vi "DropDown VI Wrapper Testing.vi"(7 "Software Config File Path":path) -> ()   [LabVIEW 2016]
uses:
  DropDown VI Wrapper Type Defs/Drop Down Bar.ctl
  <vilib>/Utility/miscctls.llb/LVPointTypeDef.ctl
  <vilib>/Utility/miscctls.llb/LVRectTypeDef.ctl
panel:
  in  "Visible Two":bool
  in  "Visible":bool
  in  "Screen and Exit Bar":T1
  in  "Drop Down Control 1":T2
  in  "Drop Down Control 2":T2
  in  "Drop Down Control 3":T2
  in  "Drop Down Control 4":T2
  in  "Drop Down Control 5":T2
  in  "Drop Down Control 6":T2
  in  "Drop Down Control 7":T2
  in  "Drop Down Control 8":T2
  in  "Drop Down Control 9":T2
  in  "Drop Down Control 10":T2
  # "Some Text"
  # "Some Text"
  # "Some Text"
  # "Some Text"
  # "Some Text"
  # "Some Text"
  # "Some Text"
  # "Some Text"
  # "Some Text"
  # "Some Text"
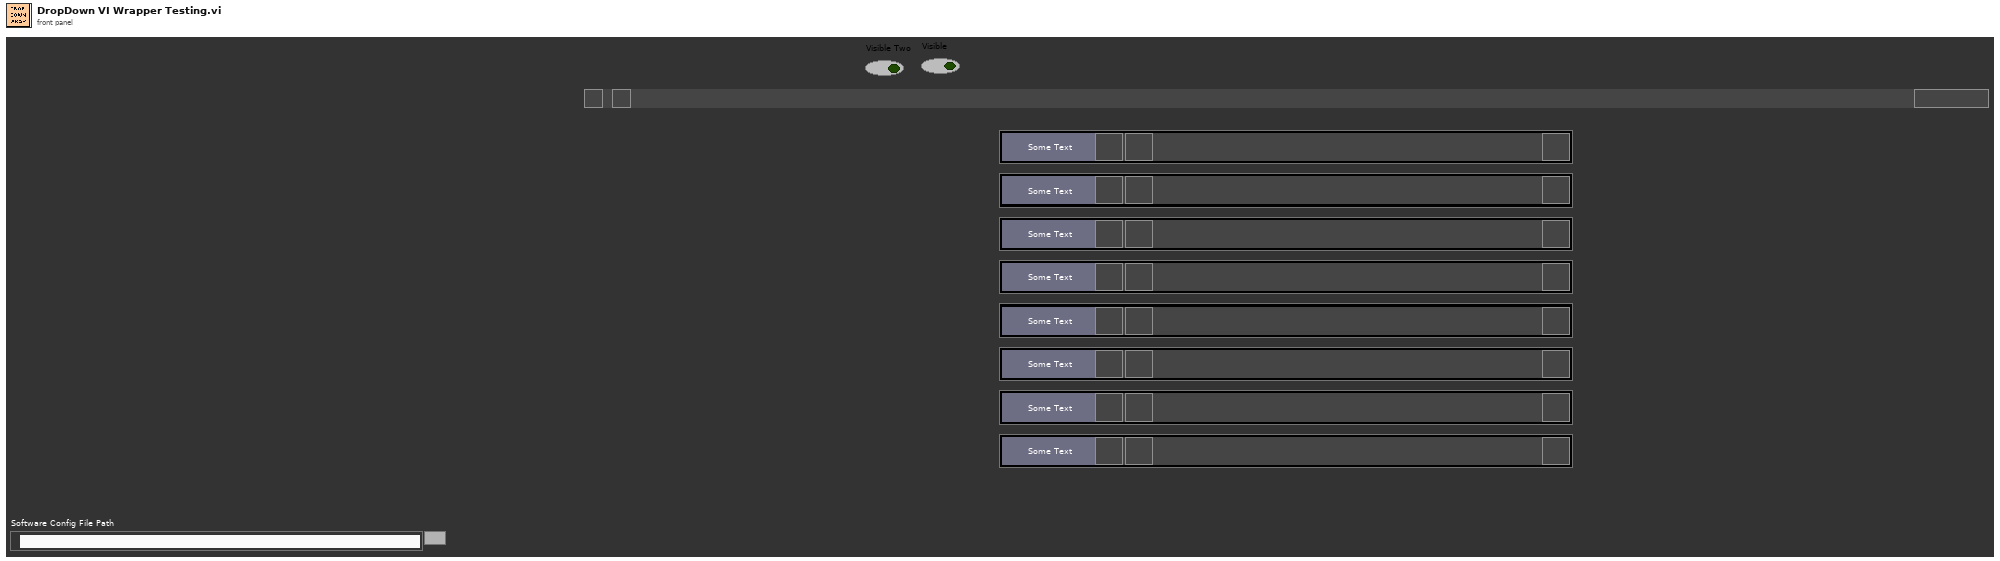
[diagram p1: front panel]
types:
  T1 = cluster{"Max Left":bool, "Max Right":bool, "Exit":bool, "Messages":string}
  T2 = typedef "Drop Down Bar.ctl" = cluster{"Right Width":bool, "Messages":string, "Abort VI":bool, "Close VI":bool}
  T3 = enum16{"Always On", "Always Off", "Off While Running"}
  T4 = typedef "LVPointTypeDef.ctl" = cluster{"Horizontal":i16, "Vertical":i16}
  T5 = enum32{"Invalid", "Standard", "Closed", "Hidden", "Minimized", "Maximized"}
  T6 = typedef "LVRectTypeDef.ctl" = cluster{"Left":i16, "Top":i16, "Right":i16, "Bottom":i16}
  T7 = enum8{"Enabled", "Disabled", "Disabled and Grayed Out"}
  T8 = cluster{"VI Path":path, "VI Refnum":refnum<vi>}[]
  T9 = typedef "lveventtype.ctl" = enum32{"Null", "Timeout", "Annotation Menu Selection", "Annotation Menu Selection?", "App Instance Close", "App Instance Close?", "Autoscale Range Change", "Bookmark Info Change", "Cell Edit", "Cell Edit?", "Cursor Grab", "Cursor Grab?", "Cursor Menu Selection", "Cursor Menu Selection?", "Cursor Move", "Cursor Release", "Data Change", "Direction Change", "Display State Change", "Drag Ended", "Drag Enter", "Drag Leave", "Drag Over", "Drag Source Update", "Drag Starting", "Drag Starting?", "Drop", "Exec State Change", "Key Down", "Key Down?", "Key Repeat", "Key Repeat?", "Key Up", "Listbox Double Click", "Menu Activation?", "Menu Selection (App)", "Menu Selection? (App)", "Menu Selection (User)", "Mouse Down", "Mouse Down?", "Mouse Enter", "Mouse Leave", "Mouse Move", "Mouse Up", "Mouse Wheel", "NI Security User Change (App)", "Pane Size", "Panel Close", "Panel Close?", "Panel Resize", "Plot Attribute Change", "Scale Range Change", "Shortcut Menu Activation?", "Shortcut Menu Selection (App)", "Shortcut Menu Selection? (App)", "Shortcut Menu Selection (User)", "Tree Double Click", "Tree Drag", "Tree Drag?", "Tree Drop", "Tree Drop?", "Tree Item Close", "Tree Item Close?", "Tree Item Open", "Tree Item Open?", "User Event", "Value Change"}
  T10 = typedef "LVAllMonitorsDisplayTypeDef.ctl" = cluster{"Bounds":cluster{"Left":i16, "Top":i16, "Right":i16, "Bottom":i16}, "Depth":i16}[]
  T11 = cluster{"Bounds":cluster{"Left":i16, "Top":i16, "Right":i16, "Bottom":i16}, "Depth":i16}
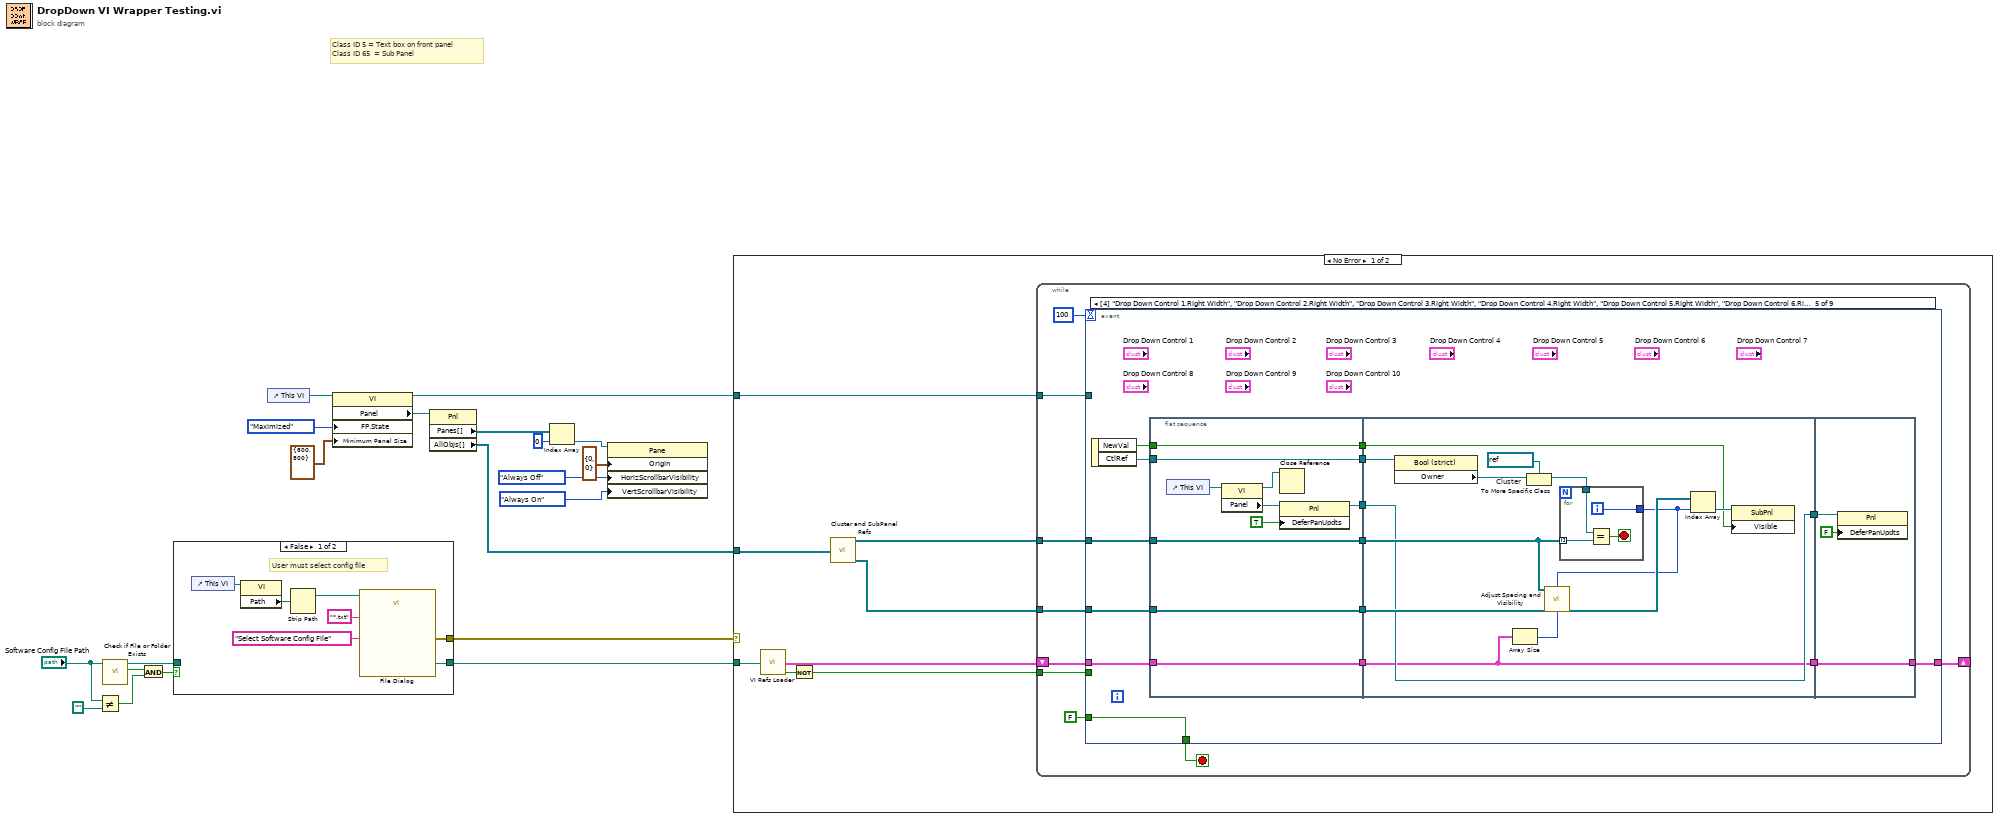
[diagram p0: block diagram]
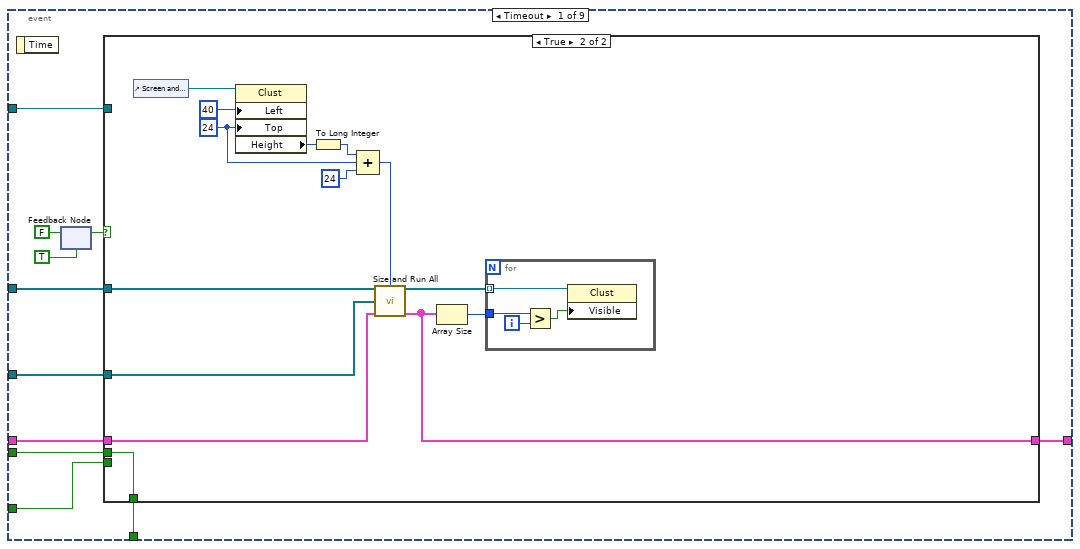
[diagram p2: hidden frame]
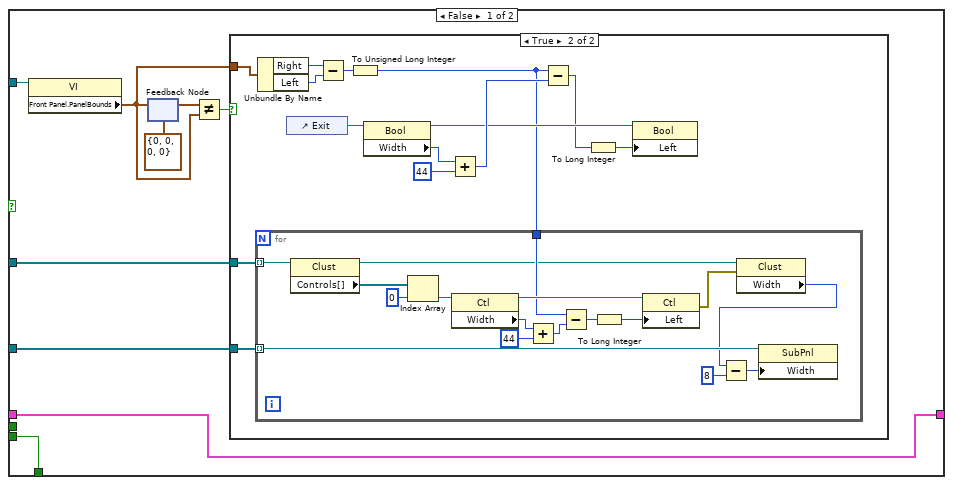
[diagram p3: hidden frame]
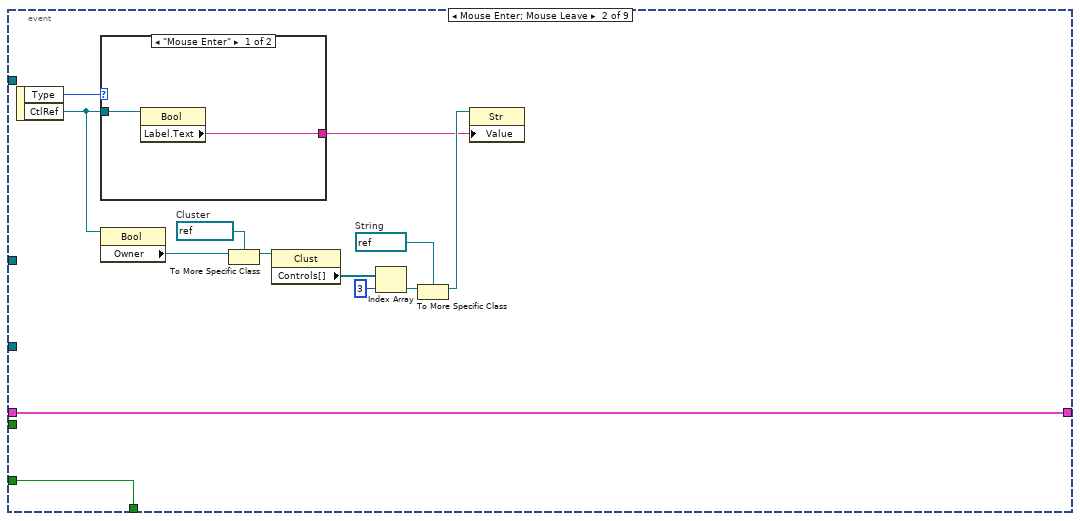
[diagram p5: hidden frame]
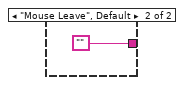
[diagram p6: hidden frame]
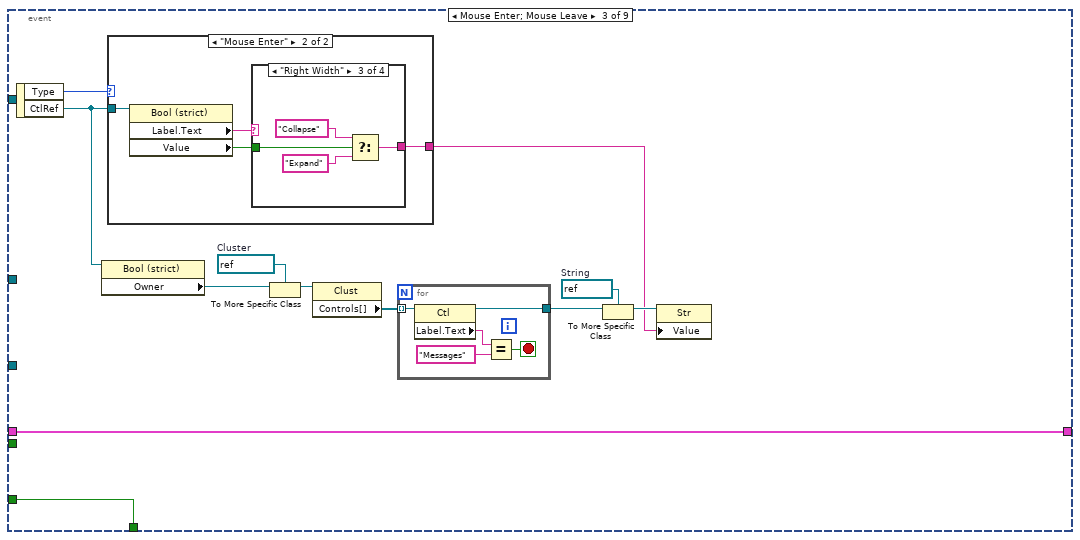
[diagram p7: hidden frame]
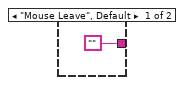
[diagram p8: hidden frame]
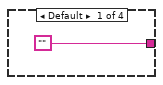
[diagram p9: hidden frame]
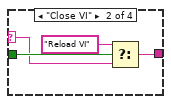
[diagram p10: hidden frame]
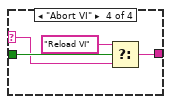
[diagram p11: hidden frame]
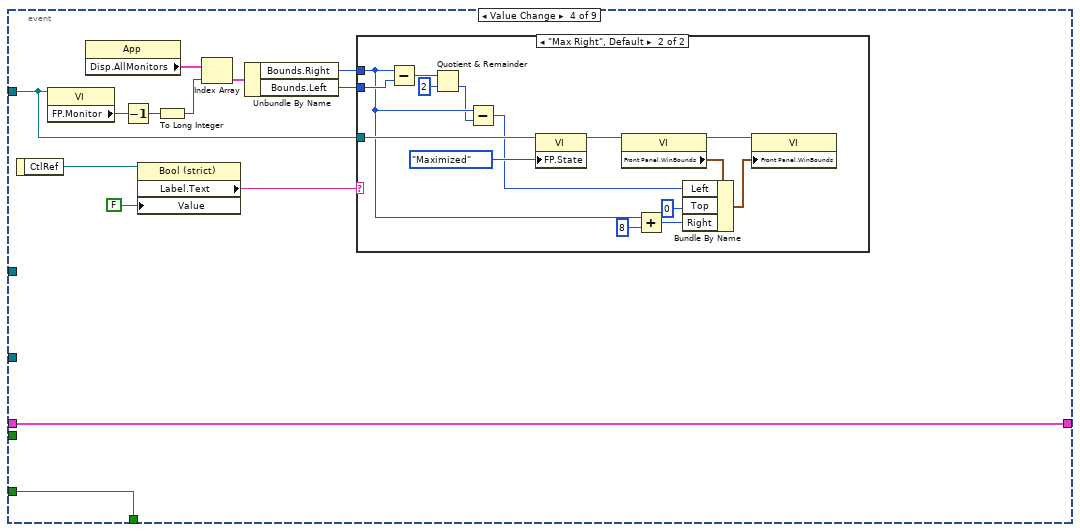
[diagram p12: hidden frame]
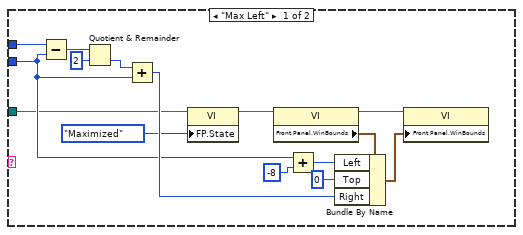
[diagram p13: hidden frame]
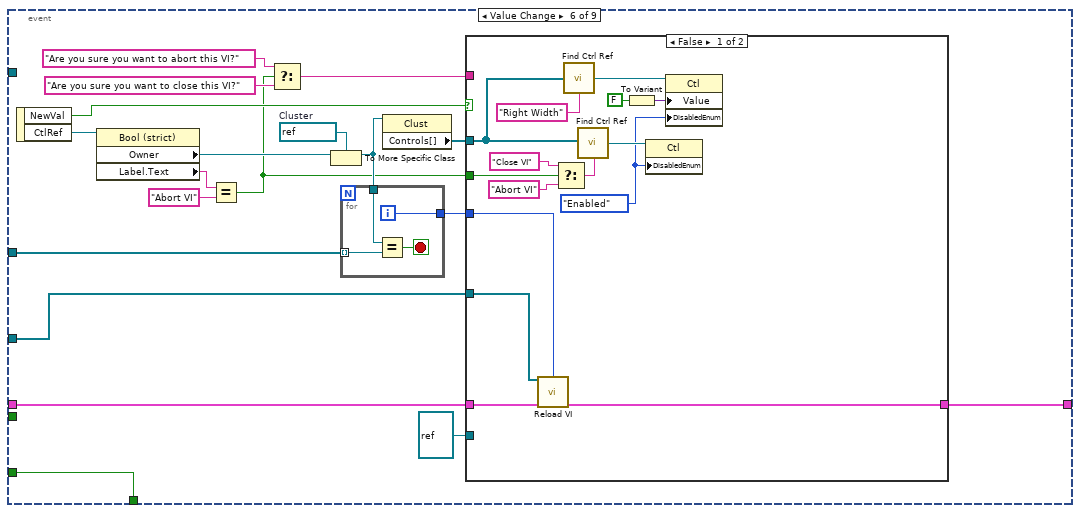
[diagram p14: hidden frame]
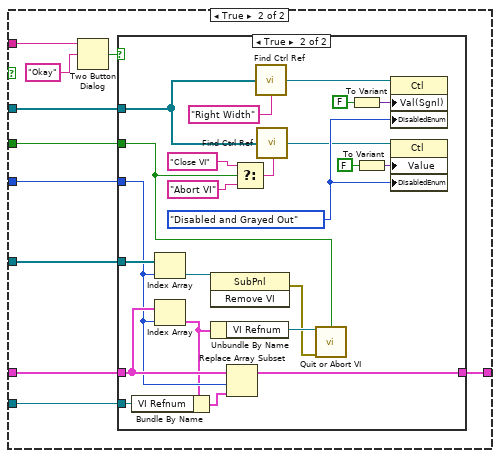
[diagram p15: hidden frame]
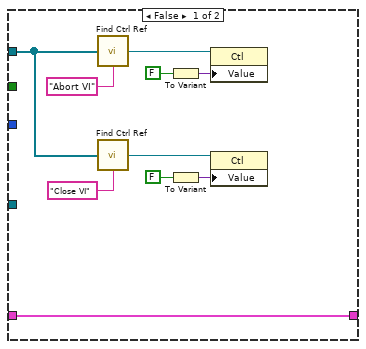
[diagram p16: hidden frame]
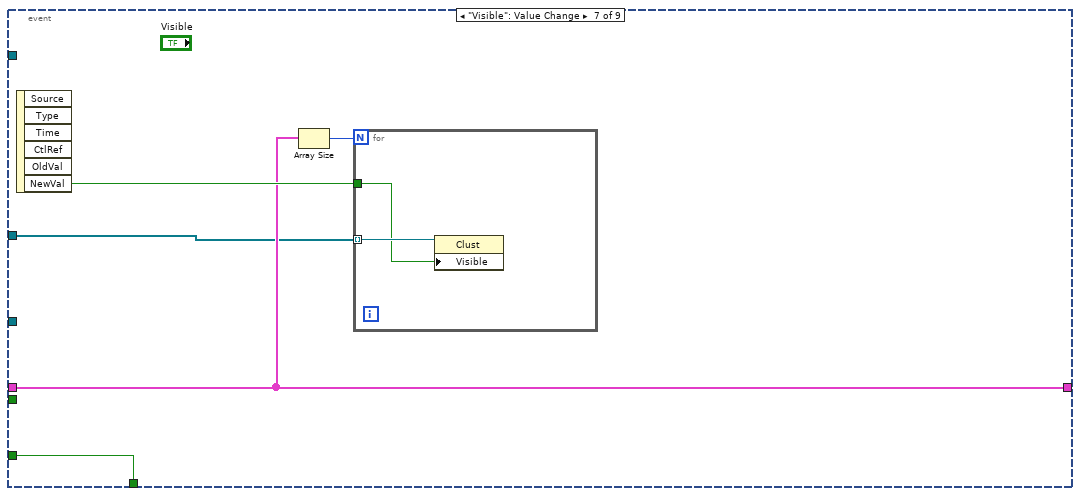
[diagram p17: hidden frame]
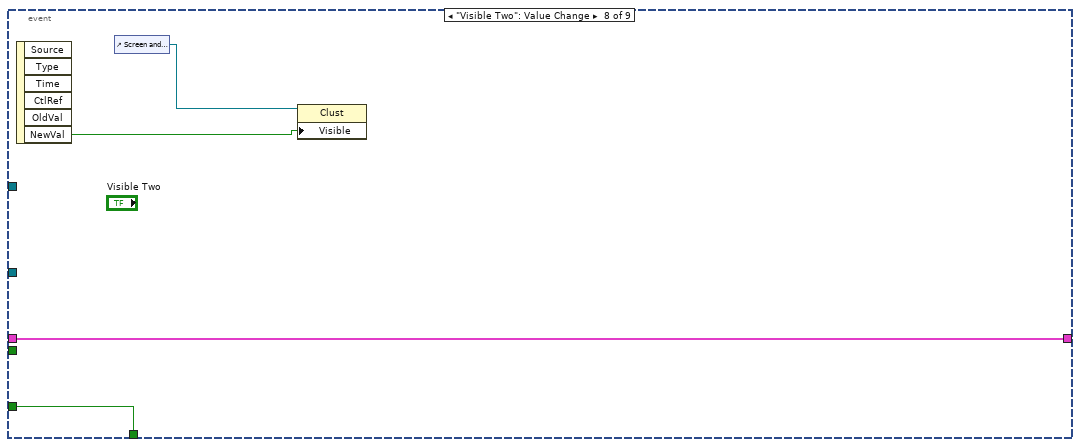
[diagram p18: hidden frame]
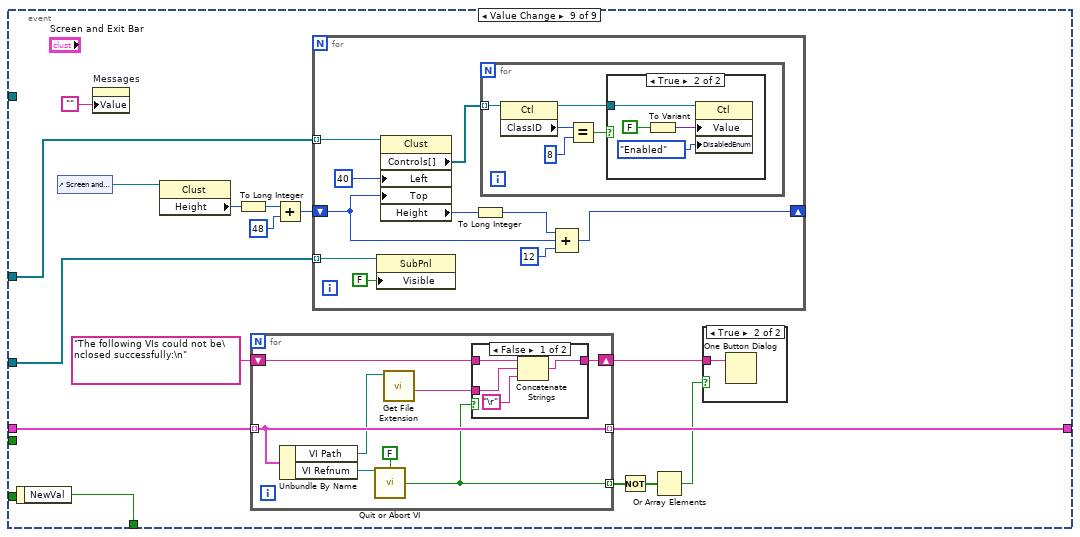
[diagram p19: hidden frame]
diagram:
  # "Class ID 5 = Text box on front panel\nClass ID 65  = Sub Panel"
  n1 = Not Equal?(x="Software Config File Path", y=path "") -> (x != y?=w7:bool)
  n2 = call <vilib>:"Check if File or Folder Exists.vi"("path"="Software Config File Path") -> ("file or folder exists?"=w6:bool, "dup path"=w4:path)  [unwired: 8 in, 1 out]
  n3 = And(x=w6, y=w7) -> (x .and. y?=w5:bool)
  n4 = case shown="False" w5 {
    tunnel: w4 -> [_ w29]
    tunnel: [w25 w29] -> w1
    tunnel: [w24 errorcluster {"status"=FALSE, "code"=0, "source"=""} ("error out")] -> w2
    frame False {
      # "User must select config file"
      n5 = control-ref of="This VI"() -> (w23:refnum<vi>)
      n6 = property class="VI"(reference=w23) -> ("Path"=w22:path)  [unwired: 1 in, 2 out]
      n7 = Strip Path(path=w22) -> (stripped path=w21:path)  [unwired: 1 out]
      n8 = call "File Dialog"("start path"=w21, "prompt"="Select Software Config File", "pattern (all files)"="*.txt") -> ("selected path"=w25:path, "error out"=w24:errorcluster)  [unwired: 9 in, 2 out]
    }
    frame True {
      # "Config File is specified - try and use it"
    }
  }
  n9 = control-ref of="This VI"() -> (w16:refnum<vi>)
  n10 = property class="VI"(reference=w16, "FP.State"=T5."Maximized" ("Front Panel Window:State"), "Minimum Panel Size"=T4 {"Horizontal"=800, "Vertical"=800} ("Front Panel Window:Minimum Size")) -> (reference out=w11:refnum<vi>, "Panel"=w10:refnum<vi>)  [unwired: 1 in, 1 out]
  n11 = property class="Pnl"(reference=w10) -> ("Panes[]"=w13:refnum<vi>[], "AllObjs[]"=w9:refnum<vi>[])  [unwired: 1 in, 2 out]
  n12 = Index Array(array=w13, index=0) -> (element=w19:refnum<vi>)
  n13 = property class="Pane"(reference=w19, "Origin"=T4 {"Horizontal"=0, "Vertical"=0}, "HorizScrollbarVisibility"=T3."Always Off" ("Vertical Scrollbar Visibility"), "VertScrollbarVisibility"=T3."Always On" ("Vertical Scrollbar Visibility")) -> ()  [unwired: 1 in, 2 out]
  n14 = case shown="No Error" w2 {
    tunnel: w11 -> [w37 _]
    tunnel: w9 -> [w35 _]
    tunnel: w1 -> [w32 _]
    frame No Error {
      n15 = call "VI Refs Loader.vi"("Config File Path"=w32) -> ("VI Path/Ref"=w34:T8, "VIs Loaded?"=w36:bool)  [unwired: 12 in, 1 out]
      n16 = Not(x=w36) -> (.not. x?=w33:bool)
      n17 = call "Cluster and SubPanel Refs.vi"("All Objects Refs"=w35) -> ("Cluster Refs"=w31:refnum<vi>[], "Sub Panel Refs"=w30:refnum<vi>[])  [unwired: 13 in]
      n18 = while {
        tunnel: w37 -> [w43]
        tunnel: w31 -> [w38]
        tunnel: w30 -> [w41]
        tunnel: w33 -> [w40]
        shift-right: [w39] -> _
        shift-left: w34 -> [w42]
        stop <- w46 stop-if-true
        n19 = event shown="[4] \"Drop Down Control 1.Right Width\", \"Drop Down Control 2.Right Width\", \"Drop Down Control 3.Right Width\", \"Drop Down Control 4.Right Width\", \"Drop Down Control 5.Right Width\", \"Drop Down Control 6.Right Width\", \"Drop Down Control 7.Right Width\", \"Drop Down Control 8.Right Width\", \"Drop Down Control 9.Right Width\", \"Drop Down Control 10.Right Width\": Value Change" {
          selector: _ -> [_ _ _ _ _ _ _ _ _]
          dyn-events: _ -> [_ _ _ _ _ _ _ _ _]
          timeout: 100 -> [_ _ _ _ _ _ _ _ _]
          tunnel: [w53 w128 w142 w179 w224 w273 w340 w346 w362] -> w46
          tunnel: FALSE -> [w52 w128 w142 w179 w224 w273 w340 w346 _]
          tunnel: w43 -> [w57 _ _ w170 _ _ _ _ _]
          tunnel: w38 -> [w56 _ _ _ w222 w268 w336 _ w360]
          tunnel: w41 -> [w55 _ _ _ w223 w266 _ _ w359]
          tunnel: w42 -> [w54 w116 w143 w167 w219 w267 w337 w345 w353]
          tunnel: w40 -> [w51 _ _ _ _ _ _ _ _]
          tunnel: [w50 w116 w143 w167 w211 w264 w337 w345 w352] -> w39
          event Timeout {
            n20 = event-data() -> ()  [unwired: 1 in, 1 out]
            n21 = feedback #1(TRUE) -> (w47:bool)
            n22 = feedback-in #1(FALSE) -> ()
            n23 = case shown="True" w47 {
              tunnel: w57 -> [w66 _]
              tunnel: w56 -> [w61 w102]
              tunnel: w55 -> [w60 w109]
              tunnel: w54 -> [w58 w108]
              tunnel: [w59 w99] -> w53
              tunnel: w52 -> [w59 _]
              tunnel: w51 -> [_ w99]
              tunnel: [w58 w98] -> w50
              frame False {
                n24 = property class="VI"(reference=w66) -> ("Front Panel.PanelBounds"=w62:T6)  [unwired: 1 in, 2 out]
                n25 = feedback-in #2(w62) -> ()
                n26 = feedback #2(T6 {"Left"=0, "Top"=0, "Right"=0, "Bottom"=0} ("Front Panel.PanelBounds")) -> (w65:T6)
                n27 = Not Equal?(x=w65, y=w62) -> (x != y?=w63:bool)
                n28 = case shown="True" w63 {
                  tunnel: w62 -> [_ w80]
                  tunnel: w61 -> [_ w70]
                  tunnel: w60 -> [_ w67]
                  frame False {
                  }
                  frame True {
                    n29 = Unbundle By Name(w80) -> ("Right"=w72:i16, "Left"=w73:i16)
                    n30 = control-ref of="Exit"() -> (w78:refnum<vi>)
                    n31 = Subtract(x=w72, y=w73) -> (x-y=w71:i16)
                    n32 = To Unsigned Long Integer(number=w71) -> (unsigned 32bit integer=w68:u32)
                    n33 = for {
                      tunnel: w70 -> [w97] mode=indexing
                      tunnel: w68 -> [w88]
                      tunnel: w67 -> [w86] mode=indexing
                      n34 = property class="Clust"(reference=w97) -> (reference out=w85:refnum<vi>, "Controls[]"=w96:refnum<vi>[])  [unwired: 1 in, 1 out]
                      n35 = Index Array(array=w96, index=0) -> (element=w92:refnum<vi>)
                      n36 = property class="Ctl"(reference=w92) -> (reference out=w91:refnum<vi>, "Width"=w93:u32)  [unwired: 1 in, 1 out]
                      n37 = Add(x=w93, y=u32 44) -> (x+y=w90:u32)
                      n38 = Subtract(x=w88, y=w90) -> (x-y=w89:u32)
                      n39 = To Long Integer(number=w89) -> (32bit integer=w94:i32)
                      n40 = property class="Ctl"(reference=w91, "Left"=w94) -> (error out=w84:errorcluster)  [unwired: 1 in, 1 out]
                      n41 = property class="Clust"(reference=w85, error in=w84) -> ("Width"=w83:u32)  [unwired: 2 out]
                      n42 = Subtract(x=w83, y=u32 8) -> (x-y=w82:u32)
                      n43 = property class="SubPnl"(reference=w86, "Width"=w82) -> ()  [unwired: 1 in, 2 out]
                    }
                    n44 = property class="Bool"(reference=w78) -> (reference out=w76:refnum<vi>, "Width"=w79:u32)  [unwired: 1 in, 1 out]
                    n45 = Add(x=w79, y=u32 44) -> (x+y=w77:u32)
                    n46 = Subtract(x=w68, y=w77) -> (x-y=w74:u32)
                    n47 = To Long Integer(number=w74) -> (32bit integer=w75:i32)
                    n48 = property class="Bool"(reference=w76, "Left"=w75) -> ()  [unwired: 1 in, 2 out]
                  }
                }
              }
              frame True {
                w106 = 24 ("Position:Top")
                n49 = control-ref of="Screen and Exit Bar"() -> (w111:refnum<vi>)
                n50 = property class="Clust"(reference=w111, "Left"=40 ("Position:Left"), "Top"=w106) -> ("Height"=w107:u32)  [unwired: 1 in, 2 out]
                n51 = To Long Integer(number=w107) -> (32bit integer=w105:i32)
                n52 = Compound Arithmetic op=ADD(w105, w106, 24 ("value")) -> (w103:i32)
                n53 = call "Size and Run All.vi"("Cluster Refs"=w102, "Initial Top Position"=w103, "Subpanel Refs"=w109, "VI Path/Ref"=w108) -> ("Cluster Refs Dup"=w101:refnum<vi>[], "VI Path/Ref Out"=w98:T8)  [unwired: 10 in]
                n54 = Array Size(array=w98) -> (size(s)=w100:i32)
                n55 = for {
                  tunnel: w101 -> [w115] mode=indexing
                  tunnel: w100 -> [w112]
                  i -> [w114]
                  n56 = Greater?(x=w112, y=w114) -> (0:w113:bool)
                  n57 = property class="Clust"(reference=w115, "Visible"=w113) -> ()  [unwired: 1 in, 2 out]
                }
              }
            }
          }
          event "Screen and Exit Bar.Exit", "Screen and Exit Bar.Max Right", "Screen and Exit Bar.Max Left": Mouse Enter; "Screen and Exit Bar.Exit", "Screen and Exit Bar.Max Right", "Screen and Exit Bar.Max Left": Mouse Leave {
            w119 = refnum<vi> refnum  # String
            w124 = refnum<vi> refnum  # Cluster
            n58 = event-data() -> ("Type"=w127:T9, "CtlRef"=w126:refnum<vi>)  [unwired: 1 in]
            n59 = case shown="\"Mouse Enter\"" w127 {
              tunnel: w126 -> [w130 _]
              tunnel: [w129 ""] -> w117
              frame "Mouse Enter" {
                n60 = property class="Bool"(reference=w130) -> ("Label.Text"=w129:string)  [unwired: 1 in, 2 out]
              }
              frame "Mouse Leave", Default {
              }
            }
            n61 = property class="Bool"(reference=w126) -> ("Owner"=w125:refnum<vi>)  [unwired: 1 in, 2 out]
            n62 = To More Specific Class(target class=w124, reference=w125) -> (specific class reference=w123:refnum<vi>)  [unwired: 1 in, 1 out]
            n63 = property class="Clust"(reference=w123) -> ("Controls[]"=w122:refnum<vi>[])  [unwired: 1 in, 2 out]
            n64 = Index Array(array=w122, index=3) -> (element=w120:refnum<vi>)
            n65 = To More Specific Class(target class=w119, reference=w120) -> (specific class reference=w118:refnum<vi>)  [unwired: 1 in, 1 out]
            n66 = property class="Str"(reference=w118, "Value"=w117) -> ()  [unwired: 1 in, 2 out]
          }
          event Mouse Enter; Mouse Leave {
            w134 = refnum<vi> refnum  # String
            w139 = refnum<vi> refnum  # Cluster
            n67 = event-data() -> ("Type"=w141:T9, "CtlRef"=w140:refnum<vi>)  [unwired: 1 in]
            n68 = property class="Bool (strict)"(reference=w140) -> ("Owner"=w137:refnum<vi>)  [unwired: 1 in, 2 out]
            n69 = case shown="\"Mouse Enter\"" w141 {
              tunnel: w140 -> [_ w153]
              tunnel: ["" w150] -> w132
              frame "Mouse Leave", Default {
              }
              frame "Mouse Enter" {
                n70 = property class="Bool (strict)"(reference=w153) -> ("Label.Text"=w152:string, "Value"=w151:bool)  [unwired: 1 in, 2 out]
                n71 = case shown="\"Right Width\"" w152 {
                  selector: w152 -> [_ w157 _ w164]
                  tunnel: w151 -> [_ w158 w162 w165]
                  tunnel: ["" w155 w159 w163] -> w150
                  frame Default {
                  }
                  frame "Close VI" {
                    n72 = Select(t="Reload VI", s=w158, f=w157) -> (s? t:f=w155:string)
                  }
                  frame "Right Width" {
                    n73 = Select(t="Collapse", s=w162, f="Expand") -> (s? t:f=w159:string)
                  }
                  frame "Abort VI" {
                    n74 = Select(t="Reload VI", s=w165, f=w164) -> (s? t:f=w163:string)
                  }
                }
              }
            }
            n75 = To More Specific Class(target class=w139, reference=w137) -> (specific class reference=w138:refnum<vi>)  [unwired: 1 in, 1 out]
            n76 = property class="Clust"(reference=w138) -> ("Controls[]"=w136:refnum<vi>[])  [unwired: 1 in, 2 out]
            n77 = for {
              tunnel: w136 -> [w148] mode=indexing
              tunnel: [w144] -> w135
              stop <- w145 stop-if-true
              n78 = property class="Ctl"(reference=w148) -> (reference out=w144:refnum<vi>, "Label.Text"=w147:string)  [unwired: 1 in, 1 out]
              n79 = Equal?(x=w147, y="Messages") -> (x = y?=w145:bool)
            }
            n80 = To More Specific Class(target class=w134, reference=w135) -> (specific class reference=w133:refnum<vi>)  [unwired: 1 in, 1 out]
            n81 = property class="Str"(reference=w133, "Value"=w132) -> ()  [unwired: 1 in, 2 out]
          }
          event "Screen and Exit Bar.Max Right", "Screen and Exit Bar.Max Left": Value Change {
            n82 = event-data() -> ("CtlRef"=w178:refnum<vi>)  [unwired: 1 in]
            n83 = property class="VI"(reference=w170) -> ("FP.Monitor"=w177:u16)  [unwired: 1 in, 2 out]
            n84 = property class="App"() -> ("Disp.AllMonitors"=w176:T10)  [unwired: 2 in, 2 out]
            n85 = Decrement(x=w177) -> (x-1=w175:u16)
            n86 = property class="Bool (strict)"(reference=w178, "Value"=FALSE) -> ("Label.Text"=w169:string)  [unwired: 1 in, 2 out]
            n87 = To Long Integer(number=w175) -> (32bit integer=w174:i32)
            n88 = Index Array(array=w176, index=w174) -> (element=w173:T11)
            n89 = Unbundle By Name(w173) -> ("Bounds.Right"=w172:i16, "Bounds.Left"=w171:i16)
            n90 = case shown="\"Max Right\", Default" w169 {
              tunnel: w172 -> [w194 w197]
              tunnel: w171 -> [w182 w201]
              tunnel: w170 -> [w180 w200]
              frame "Max Left" {
                n91 = Subtract(x=w194, y=w182) -> (x-y=w189:i16)
                n92 = Quotient & Remainder(x=w189, y=i16 2) -> (floor(x/y)=w187:i16)  [unwired: 1 out]
                n93 = Add(x=w187, y=w182) -> (x+y=w186:i16)
                n94 = property class="VI"(reference=w180, "FP.State"=T5."Maximized" ("Front Panel Window:State")) -> (reference out=w184:refnum<vi>)  [unwired: 1 in, 1 out]
                n95 = property class="VI"(reference=w184) -> (reference out=w193:refnum<vi>, "Front Panel.WinBounds"=w191:T6)  [unwired: 1 in, 1 out]
                n96 = Add(x=w182, y=i16 -8 ("Left")) -> (x+y=w181:i16)
                n97 = Bundle By Name(cluster=w191, "Left"=w181, "Top"=i16 0, "Right"=w186) -> (w192:T6)
                n98 = property class="VI"(reference=w193, "Front Panel.WinBounds"=w192) -> ()  [unwired: 1 in, 2 out]
              }
              frame "Max Right", Default {
                n99 = Subtract(x=w197, y=w201) -> (x-y=w206:i16)
                n100 = Quotient & Remainder(x=w206, y=i16 2) -> (floor(x/y)=w196:i16)  [unwired: 1 out]
                n101 = Subtract(x=w197, y=w196) -> (x-y=w195:i16)
                n102 = property class="VI"(reference=w200, "FP.State"=T5."Maximized" ("Front Panel Window:State")) -> (reference out=w203:refnum<vi>)  [unwired: 1 in, 1 out]
                n103 = property class="VI"(reference=w203) -> (reference out=w209:refnum<vi>, "Front Panel.WinBounds"=w207:T6)  [unwired: 1 in, 1 out]
                n104 = Add(x=w197, y=i16 8 ("Left")) -> (x+y=w198:i16)
                n105 = Bundle By Name(cluster=w207, "Left"=w195, "Top"=i16 0, "Right"=w198) -> (w208:T6)
                n106 = property class="VI"(reference=w209, "Front Panel.WinBounds"=w208) -> ()  [unwired: 1 in, 2 out]
              }
            }
          }
          event Value Change {
            n107 = event-data() -> ("NewVal"=w220:bool, "CtlRef"=w221:refnum<vi>)  [unwired: 1 in]
            n108 = flat-sequence {
              tunnel: w219 -> [w230]
              tunnel: w220 -> [w231]
              tunnel: w221 -> [w232]
              tunnel: w222 -> [w233]
              tunnel: w223 -> [w234]
              tunnel: [w234] -> w218
              tunnel: [w233] -> w217
              tunnel: [w232] -> w216
              tunnel: [w231] -> w215
              tunnel: [w230] -> w214
              tunnel: [w225] -> w212
              tunnel: w218 -> [w245]
              tunnel: w217 -> [w244]
              tunnel: w216 -> [w243]
              tunnel: w215 -> [w239]
              tunnel: w214 -> [w235]
              tunnel: [w236] -> w213
              tunnel: w212 -> [w236]
              tunnel: [w235] -> w210
              tunnel: w213 -> [w254]
              tunnel: [w252] -> w211
              tunnel: w210 -> [w252]
              frame #0 {
                n109 = control-ref of="This VI"() -> (w227:refnum<vi>)
                n110 = property class="VI"(reference=w227) -> (reference out=w226:refnum<vi>, "Panel"=w228:refnum<vi>)  [unwired: 1 in, 1 out]
                n111 = Close Reference(reference=w226) -> ()  [unwired: 1 in, 1 out]
                n112 = property class="Pnl"(reference=w228, "DeferPanUpdts"=TRUE ("Defer Panel Updates")) -> (reference out=w225:refnum<vi>)  [unwired: 1 in, 1 out]
              }
              frame #1 {
                w241 = refnum<vi> refnum  # Cluster
                n113 = property class="Bool (strict)"(reference=w243) -> ("Owner"=w242:refnum<vi>)  [unwired: 1 in, 2 out]
                n114 = Array Size(array=w235) -> (size(s)=w237:i32)
                n115 = To More Specific Class(target class=w241, reference=w242) -> (specific class reference=w240:refnum<vi>)  [unwired: 1 in, 1 out]
                n116 = for {
                  tunnel: w244 -> [w251] mode=indexing
                  tunnel: w240 -> [w250]
                  tunnel: [w248] -> w238
                  i -> [w248]
                  stop <- w249 stop-if-true
                  n117 = Equal?(x=w250, y=w251) -> (x = y?=w249:bool)
                }
                n118 = call "Adjust Spacing and Visibility.vi"("Cluster Ref Array"=w244, "Position Index"=w238, "Sub Panel Ref Array"=w245, "Num of VIs"=w237) -> ("Sub Panel Ref Array Dup"=w247:refnum<vi>[])  [unwired: 11 in]
                n119 = Index Array(array=w247, index=w238) -> (element=w246:refnum<vi>)
                n120 = property class="SubPnl"(reference=w246, "Visible"=w239) -> ()  [unwired: 1 in, 2 out]
              }
              frame #2 {
                n121 = property class="Pnl"(reference=w254, "DeferPanUpdts"=FALSE ("Defer Panel Updates")) -> ()  [unwired: 1 in, 2 out]
              }
            }
          }
          event Value Change {
            w271 = refnum<vi> refnum  # Cluster
            n122 = event-data() -> ("NewVal"=w265:bool, "CtlRef"=w270:refnum<vi>)  [unwired: 1 in]
            n123 = property class="Bool (strict)"(reference=w270) -> ("Owner"=w272:refnum<vi>, "Label.Text"=w262:string)  [unwired: 1 in, 2 out]
            n124 = Equal?(x=w262, y="Abort VI" ("message")) -> (x = y?=w255:bool)
            n125 = Select(t="Are you sure you want to abort this VI?" ("message"), s=w255, f="Are you sure you want to close this VI?" ("message")) -> (s? t:f=w258:string)
            n126 = To More Specific Class(target class=w271, reference=w272) -> (specific class reference=w257:refnum<vi>)  [unwired: 1 in, 1 out]
            n127 = for {
              tunnel: w268 -> [w335] mode=indexing
              tunnel: w257 -> [w334]
              tunnel: [w332] -> w269
              i -> [w332]
              stop <- w333 stop-if-true
              n128 = Equal?(x=w334, y=w335) -> (x = y?=w333:bool)
            }
            n129 = property class="Clust"(reference=w257) -> ("Controls[]"=w256:refnum<vi>[])  [unwired: 1 in, 2 out]
            n130 = case shown="False" w265 {
              tunnel: w269 -> [w285 w296]
              tunnel: w267 -> [w287 w295]
              tunnel: w266 -> [w288 w294]
              tunnel: w256 -> [w275 w290]
              tunnel: [w286 w293] -> w264
              tunnel: refnum<vi> refnum ("VI Refnum") -> [_ w292]
              tunnel: w258 -> [_ w291]
              tunnel: w255 -> [w281 w289]
              frame False {
                w274 = T7."Enabled" ("Disabled")
                n131 = call "Reload VI.vi"("Sub Panel Refs"=w288, "Index"=w285, "Path/Ref Array In"=w287) -> ("Updated Path/Ref Array"=w286:T8)  [unwired: 12 in]
                n132 = Select(t="Close VI" ("message"), s=w281, f="Abort VI" ("message")) -> (s? t:f=w282:string)
                n133 = call "Find Ctrl Ref.vi"("Control Array"=w275, "Control Label"="Right Width") -> ("Control Ref"=w278:refnum<vi>)  [unwired: 12 in, 1 out]
                n134 = call "Find Ctrl Ref.vi"("Control Array"=w275, "Control Label"=w282) -> ("Control Ref"=w280:refnum<vi>)  [unwired: 12 in, 1 out]
                n135 = To Variant(anything=FALSE) -> (Variant=w276:variant)
                n136 = property class="Ctl"(reference=w280, "DisabledEnum"=w274) -> ()  [unwired: 1 in, 2 out]
                n137 = property class="Ctl"(reference=w278, "Value"=w276, "DisabledEnum"=w274) -> ()  [unwired: 1 in, 2 out]
              }
              frame True {
                n138 = Two Button Dialog(message=w291, 2:"Okay" ("T button name (\"OK\")")) -> (T button?=w297:bool)  [unwired: 1 in]
                n139 = case shown="True" w297 {
                  tunnel: w296 -> [_ w326]
                  tunnel: w294 -> [_ w331]
                  tunnel: w295 -> [w308 w327]
                  tunnel: [w308 w324] -> w293
                  tunnel: w292 -> [_ w323]
                  tunnel: w290 -> [w302 w314]
                  tunnel: w289 -> [_ w316]
                  frame False {
                    n140 = call "Find Ctrl Ref.vi"("Control Array"=w302, "Control Label"="Abort VI") -> ("Control Ref"=w303:refnum<vi>)  [unwired: 12 in, 1 out]
                    n141 = call "Find Ctrl Ref.vi"("Control Array"=w302, "Control Label"="Close VI") -> ("Control Ref"=w301:refnum<vi>)  [unwired: 12 in, 1 out]
                    n142 = To Variant(anything=FALSE) -> (Variant=w306:variant)
                    n143 = To Variant(anything=FALSE) -> (Variant=w305:variant)
                    n144 = property class="Ctl"(reference=w303, "Value"=w306) -> ()  [unwired: 1 in, 2 out]
                    n145 = property class="Ctl"(reference=w301, "Value"=w305) -> ()  [unwired: 1 in, 2 out]
                  }
                  frame True {
                    w312 = T7."Disabled and Grayed Out" ("Disabled")
                    n146 = Index Array(array=w331, index=w326) -> (element=w330:refnum<vi>)
                    n147 = Index Array(array=w327, index=w326) -> (element=w322:cluster{"VI Path":path, "VI Refnum":refnum<vi>})
                    n148 = Bundle By Name(cluster=w322, "VI Refnum"=w323) -> (w325:cluster{"VI Path":path, "VI Refnum":refnum<vi>})
                    n149 = invoke class="SubPnl" method="Remove VI"(reference=w330) -> (error out=w317:errorcluster)  [unwired: 2 in, 2 out]
                    n150 = Unbundle By Name(w322) -> ("VI Refnum"=w318:refnum<vi>)
                    n151 = Replace Array Subset(array=w327, new element=w325, index=w326) -> (w324:T8)
                    n152 = Select(t="Close VI" ("message"), s=w316, f="Abort VI" ("message")) -> (s? t:f=w319:string)
                    n153 = call "Find Ctrl Ref.vi"("Control Array"=w314, "Control Label"="Right Width") -> ("Control Ref"=w313:refnum<vi>)  [unwired: 12 in, 1 out]
                    n154 = call "Find Ctrl Ref.vi"("Control Array"=w314, "Control Label"=w319) -> ("Control Ref"=w309:refnum<vi>)  [unwired: 12 in, 1 out]
                    n155 = call "Quit or Abort VI.vi"("VI Ref"=w318, "Abort VI?"=w316, "Error In"=w317) -> ()  [unwired: 12 in, 1 out]
                    n156 = To Variant(anything=FALSE) -> (Variant=w310:variant)
                    n157 = To Variant(anything=FALSE) -> (Variant=w329:variant)
                    n158 = property class="Ctl"(reference=w313, "Val(Sgnl)"=w310, "DisabledEnum"=w312) -> ()  [unwired: 1 in, 2 out]
                    n159 = property class="Ctl"(reference=w309, "Value"=w329, "DisabledEnum"=w312) -> ()  [unwired: 1 in, 2 out]
                  }
                }
              }
            }
          }
          event "Visible": Value Change {
            n160 = event-data() -> ("NewVal"=w339:bool)  [unwired: 1 in, 5 out]
            n161 = Array Size(array=w337) -> (size(s)=w338:i32)
            n162 = for {
              N: w338 -> [_]
              tunnel: w336 -> [w342] mode=indexing
              tunnel: w339 -> [w341]
              n163 = property class="Clust"(reference=w342, "Visible"=w341) -> ()  [unwired: 1 in, 2 out]
            }
          }
          event "Visible Two": Value Change {
            n164 = event-data() -> ("NewVal"=w343:bool)  [unwired: 1 in, 5 out]
            n165 = control-ref of="Screen and Exit Bar"() -> (w344:refnum<vi>)
            n166 = property class="Clust"(reference=w344, "Visible"=w343) -> ()  [unwired: 1 in, 2 out]
          }
          event "Screen and Exit Bar.Exit": Value Change {
            n167 = event-data() -> ("NewVal"=w362:bool)  [unwired: 1 in]
            n168 = control-ref of="Screen and Exit Bar"() -> (w356:refnum<vi>)
            n169 = property on="Messages" class="Str"("Value"="") -> ()  [unwired: 2 in, 2 out]
            n170 = property class="Clust"(reference=w356) -> ("Height"=w355:u32)  [unwired: 1 in, 2 out]
            n171 = To Long Integer(number=w355) -> (32bit integer=w357:i32)
            n172 = for {
              tunnel: w353 -> [w371] mode=indexing
              tunnel: [w371] -> w352 mode=indexing
              shift-right: [w365] -> w347
              shift-left: "The following VIs could not be\nclosed successfully:\n" -> [w366]
              tunnel: [w364] -> w350 mode=indexing
              n173 = Unbundle By Name(w371) -> ("VI Path"=w368:path, "VI Refnum"=w370:refnum<vi>)
              n174 = call "Quit or Abort VI.vi"("VI Ref"=w370, "Abort VI?"=FALSE) -> ("Close Command Successful?"=w364:bool)  [unwired: 13 in]
              n175 = call <vilib>:"Get File Extension.vi"("file"=w368) -> ("filename without extension"=w367:string)  [unwired: 6 in, 4 out]
              n176 = case shown="False" w364 {
                tunnel: w367 -> [w374 _]
                tunnel: w366 -> [w373 w376]
                tunnel: [w372 w376] -> w365
                frame False {
                  n177 = Concatenate Strings(w373, w374, "\r") -> (w372:string)
                }
                frame True {
                }
              }
            }
            n178 = Add(x=w357, y=48) -> (x+y=w354:i32)
            n179 = for {
              tunnel: w360 -> [w385] mode=indexing
              shift-right: [w384] -> _
              shift-left: w354 -> [w380]
              tunnel: w359 -> [w377] mode=indexing
              n180 = property class="SubPnl"(reference=w377, "Visible"=FALSE) -> ()  [unwired: 1 in, 2 out]
              n181 = property class="Clust"(reference=w385, "Left"=40 ("Position:Left"), "Top"=w380) -> ("Controls[]"=w379:refnum<vi>[], "Height"=w382:u32)  [unwired: 1 in, 2 out]
              n182 = To Long Integer(number=w382) -> (32bit integer=w381:i32)
              n183 = for {
                tunnel: w379 -> [w391] mode=indexing
                n184 = property class="Ctl"(reference=w391) -> (reference out=w387:refnum<vi>, "ClassID"=w390:u32)  [unwired: 1 in, 1 out]
                n185 = Equal?(x=w390, y=u32 8) -> (x = y?=w388:bool)
                n186 = case shown="True" w388 {
                  tunnel: w387 -> [_ w393]
                  frame False {
                  }
                  frame True {
                    n187 = To Variant(anything=FALSE) -> (Variant=w394:variant)
                    n188 = property class="Ctl"(reference=w393, "Value"=w394, "DisabledEnum"=T7."Enabled" ("Disabled")) -> ()  [unwired: 1 in, 2 out]
                  }
                }
              }
              n189 = Compound Arithmetic op=ADD(w381, w380, 12 ("value")) -> (w384:i32)
            }
            n190 = Not(x=w350) -> (.not. x?=w349:bool[])
            n191 = Or Array Elements(Boolean array=w349) -> (logical OR=w348:bool)
            n192 = case shown="True" w348 {
              tunnel: w347 -> [_ w363]
              frame False {
              }
              frame True {
                n193 = One Button Dialog(message=w363) -> ()  [unwired: 1 in, 1 out]
              }
            }
          }
        }
      }
    }
    frame Error {
    }
  }
